vi "DUAL GAUGE-RW Set Point.vi"(0 "Referenz in":refnum<visa-resource-name>, 1 "Setpoint":i32(ring) items=["SP 1", "SP 2", "SP 3", "SP 4"], 2 "Channel Nr.":i32(ring) items=["Channel 1", "Channel 2"], 3 "Setpoint low":dbl=1000.0 min=0.0 max=41000.0 format="%.2e", 4 "Setpoint high":dbl=1100.0 min=0.0 max=41000.0 format="%.2e", 5 "Fehler (Eingang)":errorcluster, 6 "W/R":bool) -> (14 "Referenz out":refnum<visa-resource-name>, 16 "Get Channel Nr.":i32(ring) items=["Channel 1", "Channel 2"], 17 "Get Setpoint low":dbl min=0.0 max=41000.0 format="%.2e", 18 "Get Setpoint high":dbl min=0.0 max=41000.0 format="%.2e", 19 "Cluster (Ausgang)":errorcluster)   [LabVIEW 2013, in "Dual Gauge.lvlib"]
uses:
  Dual Gauge.lvlib
panel:
  # "mbar"
  # "mbar"
  # "mbar"
  # "mbar"
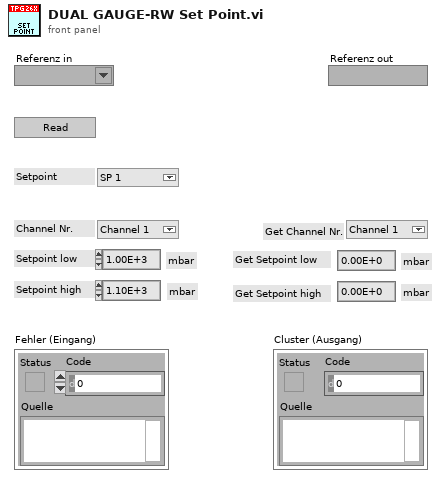
[diagram p1: front panel]
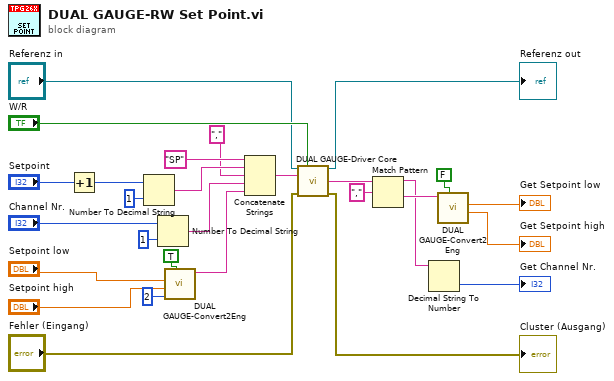
[diagram p0: block diagram]
diagram:
  n1 = Increment(x="Setpoint") -> (x+1=w23:i32)
  n2 = Number To Decimal String(number=w23, width (-)=i16 1) -> (decimal integer string=w11:string)
  n3 = Number To Decimal String(number="Channel Nr.", width (-)=i16 1) -> (decimal integer string=w13:string)
  n4 = call "DUAL GAUGE-Convert2Eng.vi"("W/R [W: Int in; Str out ]"=TRUE, "Kommastellen"=u8 2, "Eng2 in"="Setpoint high", "Eng1 in"="Setpoint low") -> ("String out"=w12:string)  [unwired: 5 in, 2 out]
  n5 = Concatenate Strings("SP" ("Command"), w11, "," ("Command"), w13, w12) -> (w5:string)
  n6 = call "DUAL GAUGE-Driver Core.vi"("Referenz in"="Referenz in", "Write/Read"="W/R", "Command"=w5, "Fehler (Eingang)"="Fehler (Eingang)") -> ("Referenz out"=→"Referenz out":refnum<visa-resource-name>, "String Out"=w8:string, "Cluster (Ausgang)"=→"Cluster (Ausgang)":errorcluster)  [unwired: 9 in]
  n7 = Match Pattern(string=w8, regular expression=",") -> (before substring=w6:string, after substring=w7:string)  [unwired: 1 in, 2 out]
  n8 = Decimal String To Number(string=w6) -> (number=→"Get Channel Nr.":i32)  [unwired: 2 in, 1 out]
  n9 = call "DUAL GAUGE-Convert2Eng.vi"("W/R [W: Int in; Str out ]"=FALSE, "String in"=w7) -> ("Eng2 out"=→"Get Setpoint high":dbl, "Eng1 out"=→"Get Setpoint low":dbl)  [unwired: 7 in, 1 out]
